vi "change bool.vi"(11 "button 6":bool) -> (3 "change arm mode":bool)   [LabVIEW 2015]
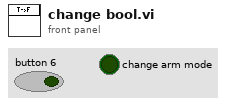
[diagram p1: front panel]
types:
  T1 = enum16{"Rising Edge", "Falling Edge", "Any Edge"}
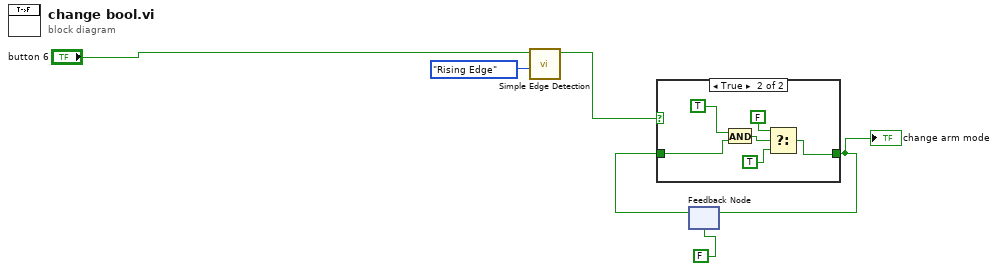
[diagram p0: block diagram]
diagram:
  n1 = call "Simple Edge Detection.vi"("Mode"=T1."Rising Edge", "clk_in"="button 6") -> ("edge?"=w4:bool)  [unwired: 9 in]
  n2 = feedback #1(FALSE) -> (w3:bool)
  n3 = case shown="True" w4 {
    tunnel: [w7 w9] -> w6
    tunnel: w3 -> [w7 w8]
    frame False {
    }
    frame True {
      n4 = And(x=TRUE, y=w8) -> (x .and. y?=w12:bool)
      n5 = Select(t=FALSE, s=w12, f=TRUE) -> (s? t:f=w9:bool)
    }
  }
  "change arm mode" <- w6
  n6 = feedback-in #1(w6) -> ()
